vi "Insert Add States.vi"(8 "error in (no error)":errorcluster, 9 "Mouse Position":T1, 10 "Variant in":path, 11 "?":refnum<vi>) -> (0 "error out":errorcluster)   [LabVIEW 2020]
doc: "Inserts the object specified by name in the Quick Drop dialog box on the selected wire(s) on the diagram. If [Shift] is also pressed, and multiple wires were selected, a single instance of the object is inserted on those wires.\n\nDefault Shortcut - [I]"
uses:
  <vilib>/Utility/miscctls.llb/LVPositionTypeDef.ctl
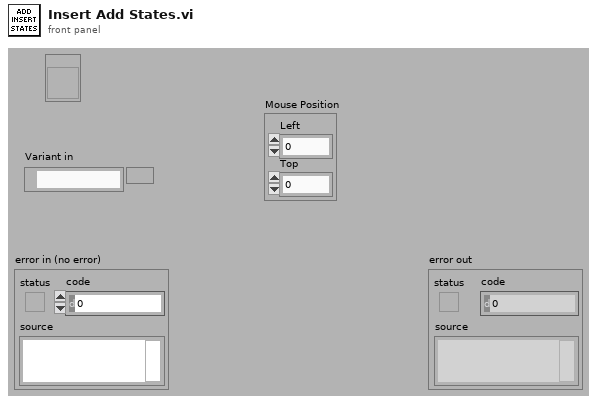
[diagram p1: front panel]
types:
  T1 = typedef "LVPositionTypeDef.ctl" = cluster{"Left":i32, "Top":i32}
  T2 = cluster{"Not Error Wire?":bool, "Source Term Top":i32, "Source Term Left":i32, "Wire Ref":refnum<vi>, "Source Term":refnum<vi>, "Sink Terms":refnum<vi>[], "Tried this one yet?":bool, "Sink Term Owner Owners":refnum<vi>[]}
  T3 = cluster{"Not Error Wire?":bool, "Source Term Top":i32, "Source Term Left":i32, "Wire Ref":refnum<vi>, "Source Term":refnum<vi>, "Sink Terms":refnum<vi>[], "Tried this one yet?":bool, "Sink Term Owner Owners":refnum<vi>[]}[]
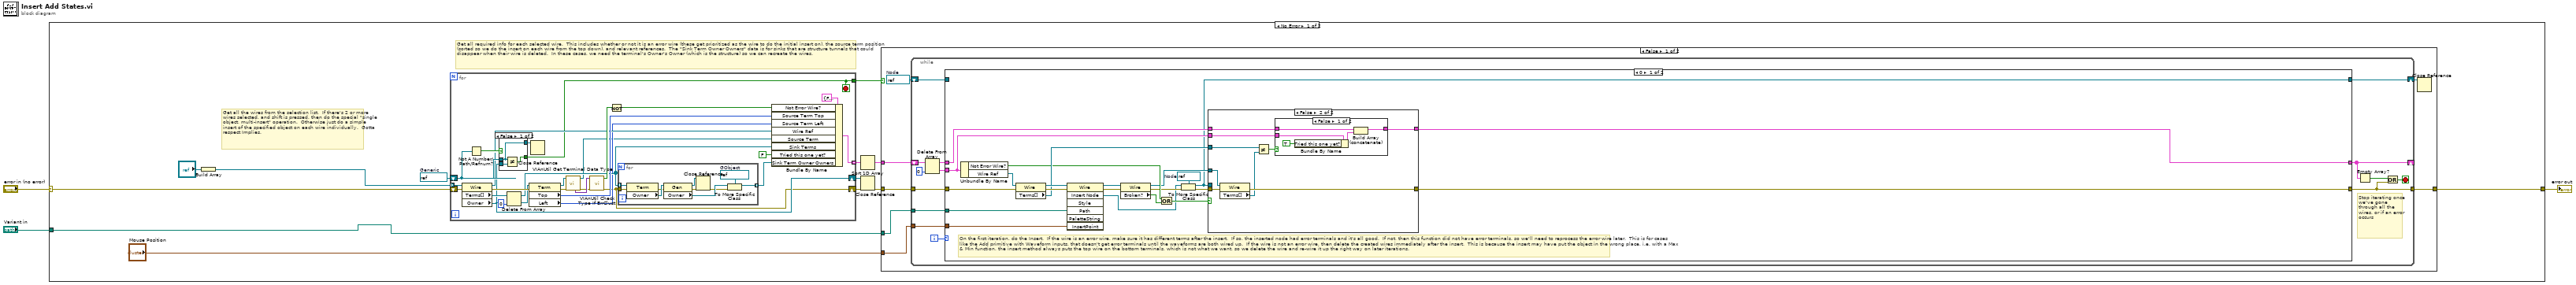
[diagram p0: block diagram]
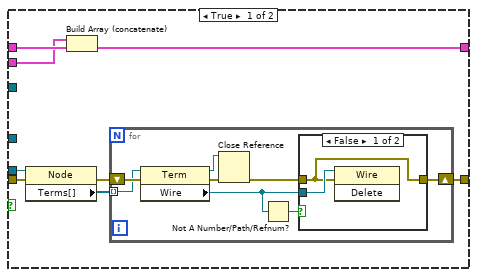
[diagram p2: hidden frame]
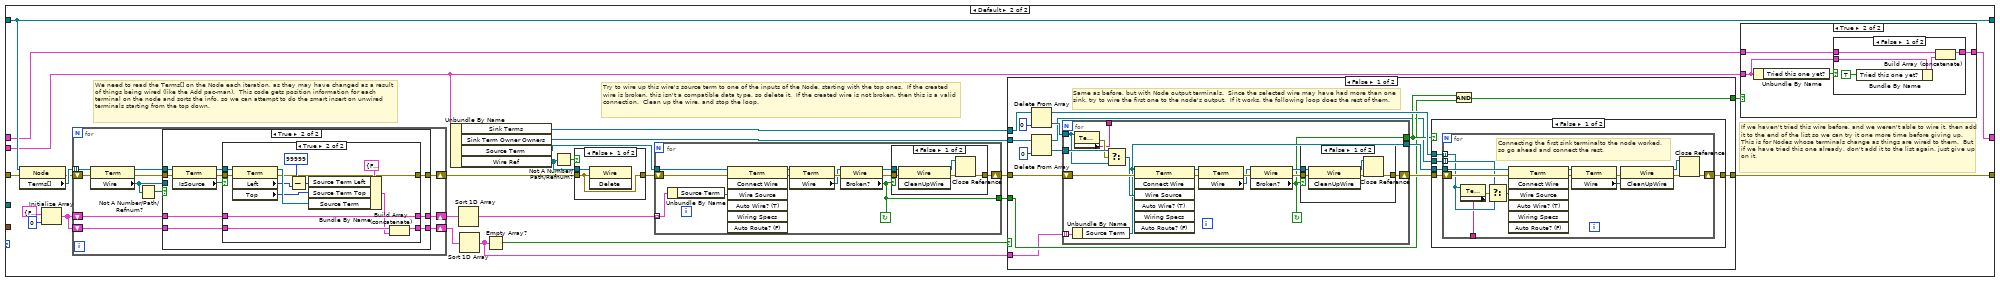
[diagram p5: hidden frame]
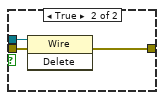
[diagram p8: hidden frame]
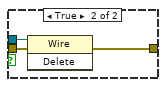
[diagram p12: hidden frame]
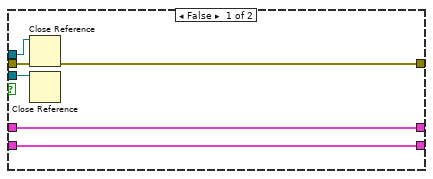
[diagram p13: hidden frame]
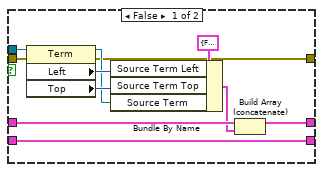
[diagram p14: hidden frame]
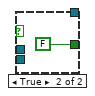
[diagram p16: hidden frame]
diagram:
  n1 = case shown="No Error" "error in (no error)" {
    selector: "error in (no error)" -> [w14 w309]
    tunnel: [w15 w309] -> w2
    tunnel: "Variant in" -> [w5 _]
    frame No Error {
      w12 = refnum<vi> refnum  # Generic
      # "Get all required info for each selected wire.  This includes whether or not it is an error wire (these get prioritized as the wire to do the initial insert on), the source term position (sorted so we do the insert on each wire from the top down), and relevant references.  The \"Sink Term Owner Owners\" data is for sinks that are structure tunnels that could disappear when their wire is deleted.  In these cases, we need the terminal's Owner's Owner (which is the structure) so we can recreate the wires."
      # "Get all the wires from the selection list.  If there's 2 or more wires selected, and shift is pressed, then do the special \"single object, multi-insert\" operation.  Otherwise just do a simple insert of the specified object on each wire individually.  Gotta respect Implies."
      n2 = Build Array("?") -> (w6:refnum<vi>[])
      n3 = for {
        shift-right: [w273] -> w8
        shift-left: w14 -> [w294]
        shift-right: [w277] -> w13
        shift-left: w12 -> [w293]
        tunnel: [w278] -> w11
        tunnel: w6 -> [w281] mode=indexing
        tunnel: [w280] -> w9 mode=indexing
        stop <- w278 stop-if-true
        n4 = property class="Wire"(reference=w281, error in=w294) -> (reference out=w284:refnum<vi>, error out=w290:errorcluster, "Terms[]"=w292:refnum<vi>[], "Owner"=w277:refnum<vi>)
        n5 = Not A Number/Path/Refnum?(number/path/refnum=w293) -> (NaN/Path/Refnum?=w289:bool)
        n6 = case shown="False" w289 {
          tunnel: [w306 FALSE] -> w278
          tunnel: w277 -> [w307 _]
          tunnel: w293 -> [w305 _]
          tunnel: [w305 _] -> w274
          frame False {
            n7 = Not Equal?(x=w305, y=w307) -> (x != y?=w306:bool)
          }
          frame True {
          }
        }
        n8 = Delete From Array(array=w292, index=0) -> (deleted portion=w279:refnum<vi>, array with subset deleted=w276:refnum<vi>[])  [unwired: 1 in]
        n9 = property class="Term"(reference=w279, error in=w290) -> (reference out=w271:refnum<vi>, error out=w272:errorcluster, "Top"=w286:i32, "Left"=w275:i32)
        n10 = Close Reference(reference=w274) -> ()  [unwired: 1 in, 1 out]
        n11 = call <vilib>:"VIAnUtil Get Terminal Data Type.vi"("error in (no error)"=w272, "Terminal in"=w271) -> ("error out"=w268:errorcluster, "Terminal out"=w270:refnum<vi>, "Type Variant"=w269:variant)  [unwired: 6 in, 1 out]
        n12 = call <vilib>:"VIAnUtil Check Type If ErrClust.vi"("error in (no error)"=w268, "Data In"=w269) -> ("error out"=w273:errorcluster, "IsErrClust?"=w287:bool)  [unwired: 8 out]
        n13 = Not(x=w287) -> (.not. x?=w285:bool)
        n14 = for {
          tunnel: w276 -> [w304] mode=indexing
          tunnel: [w301] -> w282 mode=indexing
          tunnel: w273 -> [w295]
          w300 = refnum<vi> refnum  # GObject
          n15 = property class="Term"(reference=w304, error in=w295) -> (error out=w299:errorcluster, "Owner"=w303:refnum<vi>)  [unwired: 1 out]
          n16 = property class="Gen"(reference=w303, error in=w299) -> (reference out=w297:refnum<vi>, error out=w298:errorcluster, "Owner"=w302:refnum<vi>)
          n17 = Close Reference(reference=w297, error in (no error)=w298) -> (error out=w296:errorcluster)
          n18 = To More Specific Class(target class=w300, reference=w302, error in=w296) -> (specific class reference=w301:refnum<vi>)  [unwired: 1 out]
        }
        n19 = Bundle By Name(cluster=T2 {"Not Error Wire?"=FALSE, "Source Term Top"=0, "Source Term Left"=0, "Wire Ref"=refnum, "Source Term"=refnum, "Sink Terms"=[], "Tried this one yet?"=FALSE, "Sink Term Owner Owners"=[]} ("Wire Information"), "Not Error Wire?"=w285, "Source Term Top"=w286, "Source Term Left"=w275, "Wire Ref"=w284, "Source Term"=w270, "Sink Terms"=w276, "Tried this one yet?"=FALSE, "Sink Term Owner Owners"=w282) -> (w280:T2)
      }
      n20 = Sort 1D Array(array=w9) -> (sorted array=w10:T3)
      n21 = Close Reference(reference=w13, error in (no error)=w8) -> (error out=w7:errorcluster)
      n22 = case shown="False" w11 {
        tunnel: w7 -> [w22 w267]
        tunnel: w10 -> [w23 _]
        tunnel: [w21 w267] -> w15
        tunnel: w5 -> [w18 _]
        tunnel: "Mouse Position" -> [w17 _]
        frame False {
          w20 = refnum<vi> refnum  # Node
          n23 = while {
            shift-right: [w34] -> _
            shift-left: w23 -> [w31]
            shift-right: [w26] -> w19
            shift-left: w20 -> [w33]
            tunnel: w18 -> [w27]
            tunnel: w22 -> [w35]
            tunnel: [w25] -> w21
            tunnel: w17 -> [w24]
            i -> [w36]
            stop <- w28 stop-if-true
            # "Stop iterating once we've gone through all the wires, or if an error occurs"
            n24 = Delete From Array(array=w31, index=0) -> (deleted portion=w37:T2, array with subset deleted=w30:T3)  [unwired: 1 in]
            n25 = case shown="0" w36 {
              tunnel: w37 -> [w58 w100]
              tunnel: w35 -> [w53 w119]
              tunnel: w30 -> [w45 w108]
              tunnel: [w39 w118] -> w26
              tunnel: [w59 w107] -> w34
              tunnel: w33 -> [_ w118]
              tunnel: [w57 w111] -> w25
              tunnel: w27 -> [w44 _]
              tunnel: w24 -> [w38 _]
              frame 0 {
                w42 = refnum<vi> refnum  # Node
                # "On the first iteration, do the Insert.  If the wire is an error wire, make sure it has different terms after the insert.  If so, the inserted node had error terminals and it's all good.  If not, then this function did not have error terminals, so we'll need to reprocess the error wire later.  This is for cases like the Add primitive with Waveform inputs, that doesn't get error terminals until the waveforms are both wired up.  If the wire is not an error wire, then delete the created wires immediately after the insert.  This is because the insert may have put the object in the wrong place, i.e. with a Max & Min function, the insert method always puts the top wire on the bottom terminals, which is not what we want, so we delete the wire and re-wire it up the right way on later iterations."
                n26 = Unbundle By Name(w58) -> ("Not Error Wire?"=w51:bool, "Wire Ref"=w56:refnum<vi>)
                n27 = property class="Wire"(reference=w56, error in=w53) -> (reference out=w54:refnum<vi>, error out=w55:errorcluster, "Terms[]"=w52:refnum<vi>[])
                n28 = invoke class="Wire" method="Insert Node"(reference=w54, error in=w55, "Path"=w44, "InsertPoint"=w38) -> (reference out=w50:refnum<vi>, error out=w49:errorcluster, "Insert Node"=w40:refnum<vi>)  [unwired: 3 in, 4 out]
                n29 = property class="Wire"(reference=w50, error in=w49) -> (reference out=w48:refnum<vi>, error out=w43:errorcluster, "Broken?"=w47:bool)
                n30 = Or(x=w51, y=w47) -> (x .or. y?=w46:bool)
                n31 = To More Specific Class(target class=w42, reference=w40, error in=w43) -> (specific class reference=w39:refnum<vi>, error out=w41:errorcluster)
                n32 = case shown="False" w46 {
                  tunnel: w45 -> [w67 w87]
                  tunnel: [w65 w86] -> w59
                  tunnel: w58 -> [w66 w85]
                  tunnel: [w60 w82] -> w57
                  tunnel: w41 -> [w62 w84]
                  tunnel: w48 -> [_ w83]
                  tunnel: w52 -> [_ w80]
                  tunnel: w39 -> [w63 _]
                  frame True {
                    n33 = property class="Node"(reference=w63, error in=w62) -> (error out=w64:errorcluster, "Terms[]"=w61:refnum<vi>[])  [unwired: 1 out]
                    n34 = Build Array (concatenate)(w66, w67) -> (w65:T3)
                    n35 = for {
                      shift-right: [w69] -> w60
                      shift-left: w64 -> [w75]
                      tunnel: w61 -> [w74] mode=indexing
                      n36 = property class="Term"(reference=w74, error in=w75) -> (reference out=w72:refnum<vi>, error out=w73:errorcluster, "Wire"=w68:refnum<vi>)
                      n37 = Close Reference(reference=w72, error in (no error)=w73) -> (error out=w70:errorcluster)
                      n38 = Not A Number/Path/Refnum?(number/path/refnum=w68) -> (NaN/Path/Refnum?=w71:bool)
                      n39 = case shown="False" w71 {
                        tunnel: w70 -> [w76 w78]
                        tunnel: [w76 w78] -> w69
                        tunnel: w68 -> [w77 _]
                        frame False {
                          n40 = invoke class="Wire" method="Delete"(reference=w77, error in=w76) -> ()  [unwired: 1 in, 3 out]
                        }
                        frame True {
                        }
                      }
                    }
                  }
                  frame False {
                    n41 = property class="Wire"(reference=w83, error in=w84) -> (error out=w82:errorcluster, "Terms[]"=w81:refnum<vi>[])  [unwired: 1 out]
                    n42 = Not Equal?(x=w80, y=w81) -> (x != y?=w79:bool)
                    n43 = case shown="False" w79 {
                      tunnel: w87 -> [w92 w93]
                      tunnel: [w91 w93] -> w86
                      tunnel: w85 -> [w90 _]
                      frame False {
                        n44 = Bundle By Name(cluster=w90, "Tried this one yet?"=TRUE) -> (w89:T2)
                        n45 = Build Array (concatenate)(w92, w89) -> (w91:T3)
                      }
                      frame True {
                      }
                    }
                  }
                }
              }
              frame Default {
                # "If we haven't tried this wire before, and we weren't able to wire it, then add it to the end of the list so we can try it one more time before giving up.  This is for Nodes whose terminals change as things are wired to them.  But if we have tried this one already, don't add it to the list again, just give up on it."
                # "Try to wire up this wire's source term to one of the inputs of the Node, starting with the top ones.  If the created wire is broken, this isn't a compatible data type, so delete it.  If the created wire is not broken, then this is a valid connection.  Clean up the wire, and stop the loop."
                # "We need to read the Terms[] on the Node each iteration, as they may have changed as a result of things being wired (like the Add pac-man).  This code gets position information for each terminal on the node and sorts the info, so we can attempt to do the smart insert on unwired terminals starting from the top down."
                n46 = property class="Node"(reference=w118, error in=w119) -> (error out=w116:errorcluster, "Terms[]"=w117:refnum<vi>[])  [unwired: 1 out]
                n47 = Initialize Array(T2 {"Not Error Wire?"=FALSE, "Source Term Top"=0, "Source Term Left"=0, "Wire Ref"=refnum, "Source Term"=refnum, "Sink Terms"=[], "Tried this one yet?"=FALSE, "Sink Term Owner Owners"=[]} ("Wire Information"), 0) -> (w94:T3)
                n48 = for {
                  tunnel: w117 -> [w225] mode=indexing
                  shift-right: [w218] -> w101
                  shift-left: w116 -> [w226]
                  shift-right: [w221] -> w114
                  shift-left: w94 -> [w224]
                  shift-right: [w220] -> w112
                  shift-left: w94 -> [w222]
                  n49 = property class="Term"(reference=w225, error in=w226) -> (reference out=w216:refnum<vi>, error out=w219:errorcluster, "Wire"=w217:refnum<vi>)
                  n50 = Not A Number/Path/Refnum?(number/path/refnum=w217) -> (NaN/Path/Refnum?=w223:bool)
                  n51 = case shown="True" w223 {
                    tunnel: w224 -> [w232 w239]
                    tunnel: w222 -> [w231 w238]
                    tunnel: [w232 w236] -> w221
                    tunnel: [w231 w237] -> w220
                    tunnel: w219 -> [w229 w242]
                    tunnel: [w228 w233] -> w218
                    tunnel: w217 -> [w230 _]
                    tunnel: w216 -> [w227 w241]
                    frame False {
                      n52 = Close Reference(reference=w227, error in (no error)=w229) -> (error out=w228:errorcluster)
                      n53 = Close Reference(reference=w230) -> ()  [unwired: 1 in, 1 out]
                    }
                    frame True {
                      n54 = property class="Term"(reference=w241, error in=w242) -> (reference out=w235:refnum<vi>, error out=w234:errorcluster, "IsSource"=w240:bool)
                      n55 = case shown="True" w240 {
                        tunnel: w239 -> [w252 w264]
                        tunnel: w238 -> [w253 w266]
                        tunnel: [w253 w265] -> w237
                        tunnel: [w251 w264] -> w236
                        tunnel: w235 -> [w248 w263]
                        tunnel: w234 -> [w244 w255]
                        tunnel: [w243 w254] -> w233
                        frame False {
                          n56 = property class="Term"(reference=w248, error in=w244) -> (reference out=w245:refnum<vi>, error out=w243:errorcluster, "Left"=w247:i32, "Top"=w246:i32)
                          n57 = Bundle By Name(cluster=T2 {"Not Error Wire?"=FALSE, "Source Term Top"=0, "Source Term Left"=0, "Wire Ref"=refnum, "Source Term"=refnum, "Sink Terms"=[], "Tried this one yet?"=FALSE, "Sink Term Owner Owners"=[]} ("Wire Information"), "Source Term Left"=w247, "Source Term Top"=w246, "Source Term"=w245) -> (w249:T2)
                          n58 = Build Array (concatenate)(w252, w249) -> (w251:T3)
                        }
                        frame True {
                          n59 = property class="Term"(reference=w263, error in=w255) -> (reference out=w260:refnum<vi>, error out=w254:errorcluster, "Left"=w257:i32, "Top"=w259:i32)
                          n60 = Subtract(x=99999, y=w257) -> (x-y=w256:i32)
                          n61 = Bundle By Name(cluster=T2 {"Not Error Wire?"=FALSE, "Source Term Top"=0, "Source Term Left"=0, "Wire Ref"=refnum, "Source Term"=refnum, "Sink Terms"=[], "Tried this one yet?"=FALSE, "Sink Term Owner Owners"=[]} ("Wire Information"), "Source Term Left"=w256, "Source Term Top"=w259, "Source Term"=w260) -> (w261:T2)
                          n62 = Build Array (concatenate)(w266, w261) -> (w265:T3)
                        }
                      }
                    }
                  }
                }
                n63 = Unbundle By Name(w100) -> ("Sink Terms"=w99:refnum<vi>[], "Sink Term Owner Owners"=w98:refnum<vi>[], "Source Term"=w96:refnum<vi>, "Wire Ref"=w95:refnum<vi>)
                n64 = Sort 1D Array(array=w114) -> (sorted array=w106:T3)
                n65 = Sort 1D Array(array=w112) -> (sorted array=w105:T3)
                n66 = Empty Array?(array=w105) -> (empty?=w97:bool)
                n67 = Not A Number/Path/Refnum?(number/path/refnum=w95) -> (NaN/Path/Refnum?=w104:bool)
                n68 = case shown="False" w104 {
                  tunnel: w101 -> [w120 w122]
                  tunnel: [w120 w122] -> w115
                  tunnel: w95 -> [w121 _]
                  frame False {
                    n69 = invoke class="Wire" method="Delete"(reference=w121, error in=w120) -> ()  [unwired: 1 in, 3 out]
                  }
                  frame True {
                  }
                }
                n70 = for {
                  tunnel: w96 -> [w206]
                  tunnel: w106 -> [w205] mode=indexing
                  shift-right: [w198] -> w113
                  shift-left: w115 -> [w207]
                  tunnel: [w197] -> w109
                  stop <- w197 continue-if-true
                  n71 = Unbundle By Name(w205) -> ("Source Term"=w196:refnum<vi>)
                  n72 = invoke class="Term" method="Connect Wire"(reference=w206, error in=w207, "Wire Source"=w196) -> (reference out=w203:refnum<vi>, error out=w204:errorcluster)  [unwired: 4 in, 5 out]
                  n73 = property class="Term"(reference=w203, error in=w204) -> (error out=w202:errorcluster, "Wire"=w201:refnum<vi>)  [unwired: 1 out]
                  n74 = property class="Wire"(reference=w201, error in=w202) -> (reference out=w199:refnum<vi>, error out=w200:errorcluster, "Broken?"=w197:bool)
                  n75 = case shown="False" w197 {
                    tunnel: w200 -> [w212 w214]
                    tunnel: w199 -> [w211 w215]
                    tunnel: [w208 w213] -> w198
                    frame False {
                      n76 = invoke class="Wire" method="CleanUpWire"(reference=w211, error in=w212) -> (reference out=w209:refnum<vi>, error out=w210:errorcluster)  [unwired: 1 in, 1 out]
                      n77 = Close Reference(reference=w209, error in (no error)=w210) -> (error out=w208:errorcluster)
                    }
                    frame True {
                      n78 = invoke class="Wire" method="Delete"(reference=w215, error in=w214) -> (error out=w213:errorcluster)  [unwired: 1 in, 2 out]
                    }
                  }
                }
                n79 = case shown="False" w97 {
                  tunnel: w113 -> [w138 w184]
                  tunnel: w99 -> [w137 _]
                  tunnel: [w131 w184] -> w111
                  tunnel: [w130 w183] -> w110
                  tunnel: w109 -> [w128 w183]
                  tunnel: w98 -> [w126 _]
                  tunnel: w105 -> [w123 _]
                  frame False {
                    # "Same as before, but with Node output terminals.  Since the selected wire may have had more than one sink, try to wire the first one to the node's output.  If it works, the following loop does the rest of them."
                    n80 = Delete From Array(array=w137, index=0) -> (deleted portion=w135:refnum<vi>, array with subset deleted=w132:refnum<vi>[])  [unwired: 1 in]
                    n81 = Delete From Array(array=w126, index=0) -> (deleted portion=w125:refnum<vi>, array with subset deleted=w124:refnum<vi>[])  [unwired: 1 in]
                    n82 = for {
                      tunnel: w135 -> [w160]
                      tunnel: w123 -> [w165] mode=indexing
                      shift-right: [w167] -> w134
                      shift-left: w138 -> [w174]
                      tunnel: [w162] -> w129
                      tunnel: [w163] -> w133
                      tunnel: w125 -> [w166]
                      tunnel: [w159] -> _
                      stop <- w162 continue-if-true
                      n83 = Unbundle By Name(w165) -> ("Source Term"=w163:refnum<vi>)
                      n84 = property class="Term"(reference=w160) -> (error out=w161:errorcluster, "ClassName"=w159:string)  [unwired: 1 in, 1 out]
                      n85 = Select(t=w166, s=w161, f=w160) -> (s? t:f=w164:refnum<vi>)
                      n86 = invoke class="Term" method="Connect Wire"(reference=w163, error in=w174, "Wire Source"=w164) -> (reference out=w172:refnum<vi>, error out=w173:errorcluster)  [unwired: 4 in, 5 out]
                      n87 = property class="Term"(reference=w172, error in=w173) -> (error out=w171:errorcluster, "Wire"=w170:refnum<vi>)  [unwired: 1 out]
                      n88 = property class="Wire"(reference=w170, error in=w171) -> (reference out=w168:refnum<vi>, error out=w169:errorcluster, "Broken?"=w162:bool)
                      n89 = case shown="False" w162 {
                        tunnel: w169 -> [w179 w181]
                        tunnel: w168 -> [w178 w182]
                        tunnel: [w175 w180] -> w167
                        frame False {
                          n90 = invoke class="Wire" method="CleanUpWire"(reference=w178, error in=w179) -> (reference out=w176:refnum<vi>, error out=w177:errorcluster)  [unwired: 1 in, 1 out]
                          n91 = Close Reference(reference=w176, error in (no error)=w177) -> (error out=w175:errorcluster)
                        }
                        frame True {
                          n92 = invoke class="Wire" method="Delete"(reference=w182, error in=w181) -> (error out=w180:errorcluster)  [unwired: 1 in, 2 out]
                        }
                      }
                    }
                    n93 = case shown="False" w129 {
                      tunnel: w134 -> [w143 w158]
                      tunnel: [w140 w158] -> w131
                      tunnel: w133 -> [w142 _]
                      tunnel: w132 -> [w141 _]
                      tunnel: w124 -> [w139 _]
                      frame False {
                        n94 = for {
                          tunnel: w142 -> [w156]
                          tunnel: w141 -> [w145] mode=indexing
                          shift-right: [w149] -> w140
                          shift-left: w143 -> [w157]
                          tunnel: w139 -> [w148] mode=indexing
                          tunnel: [w144] -> _
                          # "Connecting the first sink terminalto the node worked, so go ahead and connect the rest."
                          n95 = property class="Term"(reference=w145) -> (error out=w146:errorcluster, "ClassName"=w144:string)  [unwired: 1 in, 1 out]
                          n96 = Select(t=w148, s=w146, f=w145) -> (s? t:f=w147:refnum<vi>)
                          n97 = invoke class="Term" method="Connect Wire"(reference=w156, error in=w157, "Wire Source"=w147) -> (reference out=w155:refnum<vi>, error out=w154:errorcluster)  [unwired: 4 in, 5 out]
                          n98 = property class="Term"(reference=w155, error in=w154) -> (error out=w153:errorcluster, "Wire"=w152:refnum<vi>)  [unwired: 1 out]
                          n99 = invoke class="Wire" method="CleanUpWire"(reference=w152, error in=w153) -> (reference out=w150:refnum<vi>, error out=w151:errorcluster)  [unwired: 1 in, 1 out]
                          n100 = Close Reference(reference=w150, error in (no error)=w151) -> (error out=w149:errorcluster)
                        }
                      }
                      frame True {
                        # "None of the node outputs would connect to this wire.  No need to try to process the rest of the sinks."
                      }
                    }
                    n101 = And(x=w129, y=w128) -> (x .and. y?=w130:bool)
                  }
                  frame True {
                    # "There are no more unwired outputs on the node.  Don't bother trying to find one to wire to."
                  }
                }
                n102 = case shown="True" w110 {
                  tunnel: w108 -> [w185 w189]
                  tunnel: w100 -> [_ w186]
                  tunnel: [w185 w187] -> w107
                  frame False {
                  }
                  frame True {
                    n103 = Unbundle By Name(w186) -> ("Tried this one yet?"=w188:bool)
                    n104 = case shown="False" w188 {
                      tunnel: w189 -> [w194 w195]
                      tunnel: [w193 w195] -> w187
                      tunnel: w186 -> [w192 _]
                      frame False {
                        n105 = Bundle By Name(cluster=w192, "Tried this one yet?"=TRUE) -> (w191:T2)
                        n106 = Build Array (concatenate)(w194, w191) -> (w193:T3)
                      }
                      frame True {
                      }
                    }
                  }
                }
              }
            }
            n107 = Empty Array?(array=w34) -> (empty?=w29:bool)
            n108 = Or(x=w29, y=w25) -> (x .or. y?=w28:bool)
          }
          n109 = Close Reference(reference=w19) -> ()  [unwired: 1 in, 1 out]
        }
        frame True {
          # "The wires weren't all on the same diagram.  This is a no-op."
        }
      }
    }
    frame Error {
    }
  }
  "error out" <- w2
